vi "AscriptStepsToText.vi"(11 "AutoScriptSteps":T1(array[cluster])) -> (3 "AscriptLines":string[](array[string]))   [LabVIEW 2015]
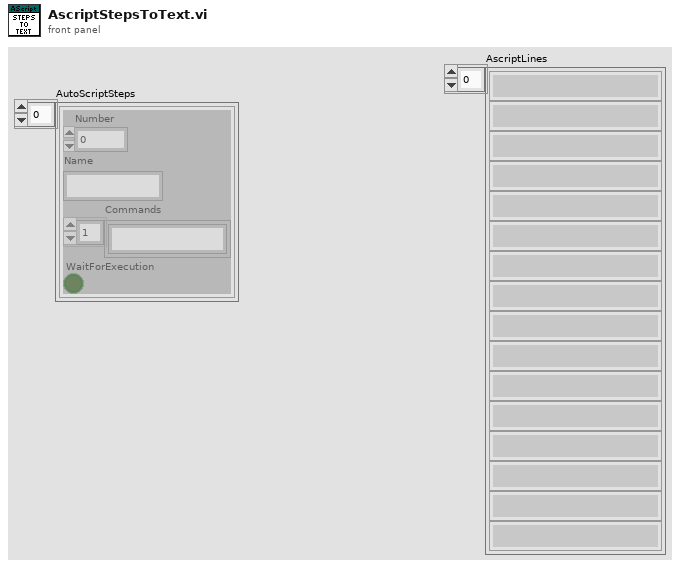
[diagram p1: front panel]
types:
  T1 = cluster{"Number":i32, "Name":string, "Commands":string[], "WaitForExecution":bool}[]
  T2 = cluster{"Return Variable Names":refnum<vi>, "ArgumentsBox":refnum<vi>, "Routine":refnum<vi>, "AddCmd":refnum<vi>, "ClearSteps":refnum<vi>, "AddStep":refnum<vi>, "DeleteAuto":refnum<vi>, "DeleteCommand":refnum<vi>, "DeleteStep":refnum<vi>, "TemplateOpen":refnum<vi>, "SaveStep":refnum<vi>, "LoadAuto":refnum<vi>, "SaveAuto":refnum<vi>, "LoadStep":refnum<vi>, "AutoFiles":refnum<vi>, "DeleteLog":refnum<vi>, "GetLogFile":refnum<vi>, "Auto Script on Robot":refnum<vi>, "DLfromRIO":refnum<vi>, "Autoscript Layout":refnum<vi>, "Auto Script Name":refnum<vi>, "ULtoRIO":refnum<vi>}
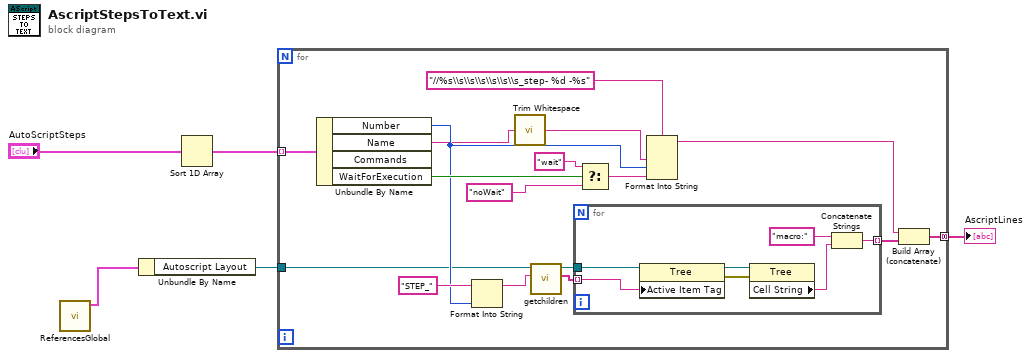
[diagram p0: block diagram]
diagram:
  n1 = call "ReferencesGlobal.vi"() -> ("AscriptRefsOut"=w1:T2)  [unwired: 11 in]
  n2 = Unbundle By Name(w1) -> ("Autoscript Layout"=w2:refnum<vi>)
  n3 = Sort 1D Array(array="AutoScriptSteps") -> (sorted array=w4:T1)
  n4 = for {
    tunnel: w4 -> [w22] mode=indexing
    tunnel: [w19] -> w3 mode=concatenating
    tunnel: w2 -> [w11]
    n5 = Unbundle By Name(w22) -> ("Number"=w13:i32, "Name"=w7:string, "WaitForExecution"=w18:bool)  [unwired: 1 out]
    n6 = Format Into String(initial string="STEP_", w13) -> (resulting string=w12:string)  [unwired: 2 in, 1 out]
    n7 = call <vilib>:"Trim Whitespace.vi"("string"=w7) -> ("trimmed string"=w6:string)  [unwired: 1 in]
    n8 = call "getchildren.vi"("Parent Tag"=w12, "Tree Reference In"=w11) -> ("Children Tags"=w10:string[], "Tree Reference Out"=w8:refnum<vi>)  [unwired: 7 in, 1 out]
    n9 = for {
      tunnel: w10 -> [w26] mode=indexing
      tunnel: [w28] -> w9 mode=indexing
      tunnel: w8 -> [w27]
      n10 = property class="Tree"(reference=w27, "Active Item Tag"=w26) -> (reference out=w25:refnum<vi>, error out=w24:errorcluster)  [unwired: 1 in]
      n11 = property class="Tree"(reference=w25, error in=w24) -> ("Cell String"=w23:string)  [unwired: 2 out]
      n12 = Concatenate Strings("macro:" ("string"), w23) -> (w28:string)
    }
    n13 = Select(t="wait", s=w18, f="noWait") -> (s? t:f=w16:string)
    n14 = Format Into String(format string="//%s\\s\\s\\s\\s\\s\\s_step- %d -%s", w6, w13, w16) -> (resulting string=w20:string)  [unwired: 2 in, 1 out]
    n15 = Build Array (concatenate)(w20, w9) -> (w19:string[])
  }
  "AscriptLines" <- w3
